vi "Subscribe.vi"(5 "Caller Enqueuer":refnum<class "Message Enqueuer.lvclass">, 7 "Self Enqueuer":refnum<class "Message Enqueuer.lvclass">, 8 "error in (no error)":errorcluster, 9 "Pre-preocess datasockets":bool, 10 "Topics":string[](array[string])=["Result"], 11 "Response Synchronizer in":refnum<class "Response Synchronizer.lvclass">) -> (0 "error out":errorcluster, 3 "Response Synchronizer out":refnum<class "Response Synchronizer.lvclass">)   [LabVIEW 2021, in "Response Synchronizer.lvclass"]
uses:
  Response Synchronizer.lvclass
  <vilib>/ActorFramework/Message Enqueuer/Message Enqueuer.lvclass
  Publish-Subscribe/Context.ctl
  Publish-Subscribe/Interfaces/Publisher Messages/Subscribe Msg/Subscribe Msg.lvclass/Subscribe Msg.ctl
  <vilib>/ActorFramework/Message Enqueuer/Message Enqueuer.lvclass/Message Enqueuer.ctl
  <vilib>/ActorFramework/Message Enqueuer/Enqueue.vi
  Publish-Subscribe/Interfaces/Publisher Messages/Subscribe Msg/Subscribe Msg.lvclass
  C:/Program Files/National Instruments/LabVIEW 2021/vi.lib/ActorFramework/Message/Message.lvclass
  <vilib>/ActorFramework/Message Priority Queue/Priority Enqueue.vi
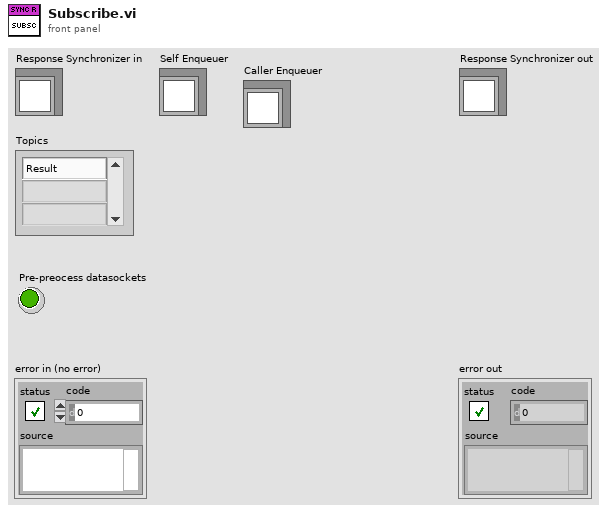
[diagram p1: front panel]
types:
  T1 = typedef "Context.ctl" = cluster{"Topic":string, "Source":string}
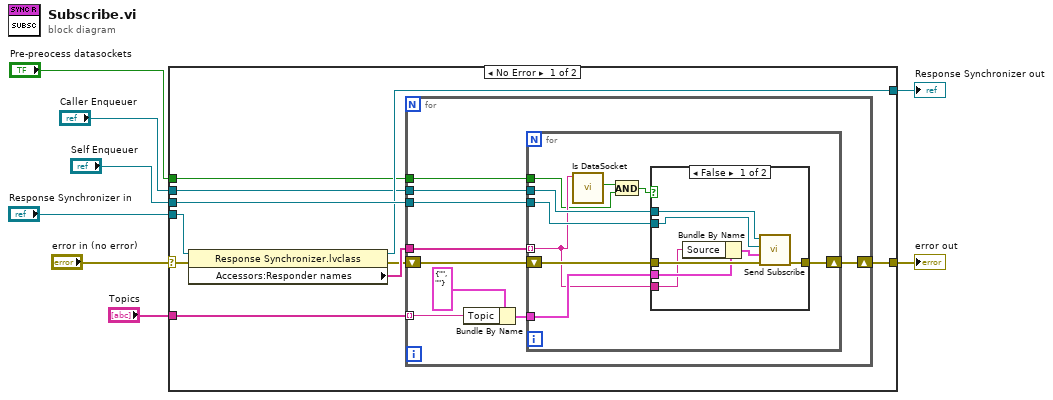
[diagram p0: block diagram]
diagram:
  n1 = case shown="No Error" "error in (no error)" {
    selector: "error in (no error)" -> [w11 w46]
    tunnel: [w16 w46] -> w7
    tunnel: [w14 w45] -> w5
    tunnel: "Response Synchronizer in" -> [w18 w45]
    tunnel: "Self Enqueuer" -> [w17 _]
    tunnel: "Topics" -> [w15 _]
    tunnel: "Caller Enqueuer" -> [w12 _]
    tunnel: "Pre-preocess datasockets" -> [w9 _]
    frame No Error {
      n2 = property class="Response Synchronizer.lvclass"(reference=w18, error in=w11) -> (reference out=w14:refnum<class "Response Synchronizer.lvclass">, error out=w10:errorcluster, "Accessors:Responder names"=w13:string[])
      n3 = for {
        tunnel: w17 -> [w27]
        tunnel: w15 -> [w23] mode=indexing
        tunnel: w13 -> [w22]
        tunnel: w12 -> [w21]
        tunnel: w9 -> [w19]
        shift-right: [w26] -> w16
        shift-left: w10 -> [w20]
        n4 = Bundle By Name(cluster=T1 {"Topic"="", "Source"=""} ("Context"), "Topic"=w23) -> (w24:T1)
        n5 = for {
          tunnel: w22 -> [w31] mode=indexing
          tunnel: w21 -> [w34]
          tunnel: w27 -> [w36]
          tunnel: w24 -> [w32]
          shift-right: [w33] -> w26
          shift-left: w20 -> [w35]
          tunnel: w19 -> [w28]
          n6 = call "Is DataSocket.vi"("String"=w31) -> ("DataSocket"=w29:bool)  [unwired: 9 in, 1 out]
          n7 = And(x=w29, y=w28) -> (x .and. y?=w30:bool)
          n8 = case shown="False" w30 {
            tunnel: w36 -> [w43 _]
            tunnel: w35 -> [w42 w44]
            tunnel: w34 -> [w40 _]
            tunnel: [w39 w44] -> w33
            tunnel: w32 -> [w38 _]
            tunnel: w31 -> [w37 _]
            frame False {
              n9 = Bundle By Name(cluster=w38, "Source"=w37) -> (w41:T1)
              n10 = call "Send Subscribe.vi"("error in (no error)"=w42, "Context"=w41, "Subscriber Enq"=w43, "Message Enqueuer"=w40) -> ("error out"=w39:errorcluster)  [unwired: 6 in, 1 out]
            }
            frame True {
            }
          }
        }
      }
    }
    frame Error {
    }
  }
  "error out" <- w7
  "Response Synchronizer out" <- w5
